vi "Create.vi"(10 "Node":refnum<class "Node.lvclass">) -> (3 "VolatusNodeValue out":refnum<class "VolatusNodeValue.lvclass">)   [LabVIEW 2020, in "Volatus.lvlib" / "VolatusNodeValue.lvclass"]
uses:
  VolatusNodeValue.lvclass
  VolatusNodeValue.lvclass/VolatusNodeValue.ctl
  VolatusConfig/Node/Node.lvclass
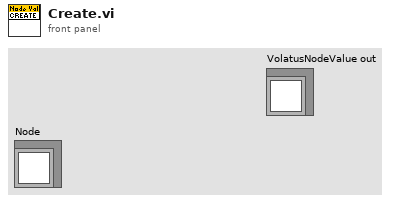
[diagram p1: front panel]
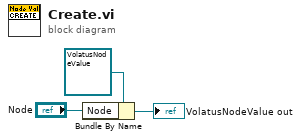
[diagram p0: block diagram]
diagram:
  n1 = Bundle By Name(cluster=refnum<class "VolatusNodeValue.lvclass"> refnum ("VolatusNodeValue in"), "Node"="Node") -> (→"VolatusNodeValue out":refnum<class "VolatusNodeValue.lvclass">)
